vi "GetEndpointInfo.vi"(7 "LabVIEW Web Service Request":refnum<class "Web Request.lvclass">) -> ()   [LabVIEW 2017]
uses:
  <vilib>/wsapi/Web Request.lvclass
  JsonableWirelessEndpoint.ctl
  JsonableWirelessChannel.ctl
  <vilib>/addons/InsightCM/Devices/Shared/Ble/BleComm/BleComm.lvlib
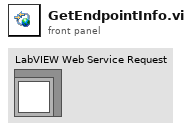
[diagram p1: front panel]
types:
  T1 = typedef "BleComm.lvlib/Endpoint.ctl" = cluster{"Serial Number":u64, "Ble Address":string, "Endpoint Type":T2, "Firmware Version":string, "Ignore Firmware":bool, "Firmware Recovery Mode":bool, "Password":string, "New Password":string, "Config Version":i32, "Sensor Group Id":string, "State":T3, "Acquiring":bool, "Acquisition Start Time":timestamp, "Ignore Gate":bool, "Sample Rate":T4, "Samples to Read":u32, "Last Communication":timestamp, "Last Acquisition":timestamp, "State Change":timestamp, "Last Status":timestamp, "Endpoint Busy Count":i32, "Properties":T5[], "Channels":T6[], "Gate":T7, "Error Timestamps":timestamp[]}
  T2 = typedef "BleComm.lvlib/Type.ctl" = enum16{"Gateway", "Spider", "Bluenose"}
  T3 = typedef "BleComm.lvlib/EndpointState.ctl" = enum16{"Unknown", "Discovered", "Bond Requested", "Bonded", "Firmware Version Requested", "Firmware Version Received", "Firmware Update Requested", "Firmware Ok", "Change Password Requested", "Password Ok", "Radio Update Requested", "Radio Ok", "Configure Requested", "Configured", "Error", "Error - Unbonding", "Error - Unknown", "Error - Quarantined"}
  T4 = typedef "Bluetooth Sensing.lvlib/SampleRate.ctl" = enum16{"25.6 kHz", "12.8 kHz", "6.4 kHz", "3.2 kHz", "1.6 kHz", "800 Hz"}
  T5 = typedef "KeyValuePair.ctl" = cluster{"Key":string, "Value":string}
  T6 = typedef "BleComm.lvlib/WirelessChannel.ctl" = cluster{"Channel Number":i32, "AssetId":string, "Sensor Type":string, "Mode":enum16{"Off", "Averaged", "Waveform"}, "Sensitivity":dbl, "Offset":dbl, "IEPE":enum16{"4 mA", "3 mA", "Off", "2 mA"}, "Coupling":enum16{"AC w/10 Hz cutoff", "AC w/2 Hz cutoff", "DC"}, "Unit":string, "Sw Ac Coupling":bool}
  T7 = typedef "BleComm.lvlib/Gate.ctl" = cluster{"Channel":u8, "Feature":string, "Level (EU)":dbl, "Properties":variant}
  T8 = typedef "JsonableWirelessEndpoint.ctl" = cluster{"Serial Number":string, "State":string, "Ble address":string, "Endpoint Type":string, "Firmware Version":string, "Password":string, "New Password":string, "Config Version":i32, "Sensor Group Id":string, "Acquisition Start Time":string, "Last Communication":string, "Last Acquisition":string, "State Change":string, "Endpoint Busy Count":i32, "Sample Rate":string, "Samples to Read":u32, "Properties":cluster{"Key":string, "Value":string}[], "Channels":T9[], "Gate Channel":u8, "Gate Feature":string, "Gate Level (EU)":dbl, "Error Timestamps":string[]}
  T9 = typedef "JsonableWirelessChannel.ctl" = cluster{"Channel Number":i32, "Type":string, "Sensitivity":dbl, "Offset":dbl, "IEPE":string, "Coupling":string, "Unit":string, "Sw Ac Coupling":bool}
  T10 = enum16{"AC w/10 Hz cutoff", "AC w/2 Hz cutoff", "DC"}
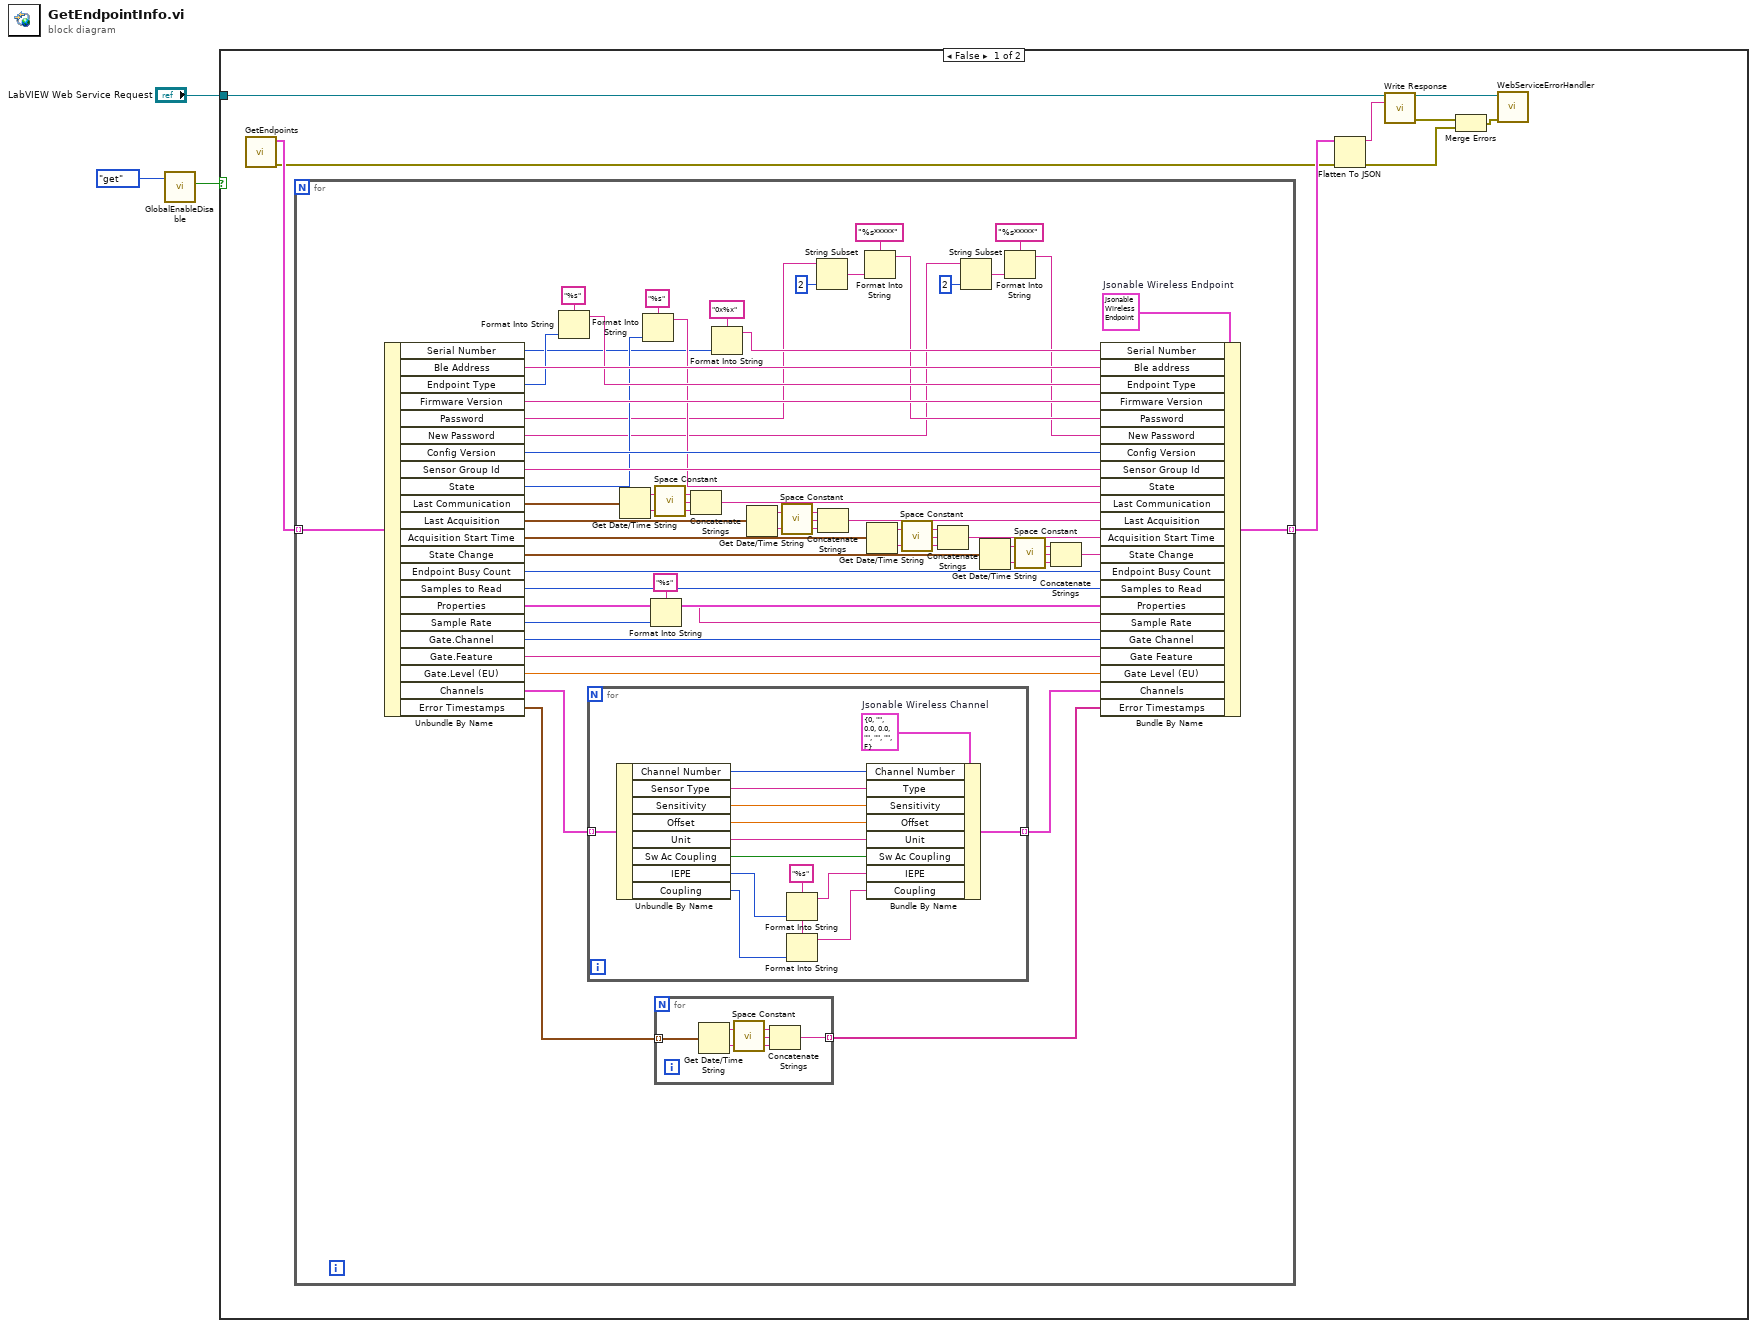
[diagram p0: block diagram]
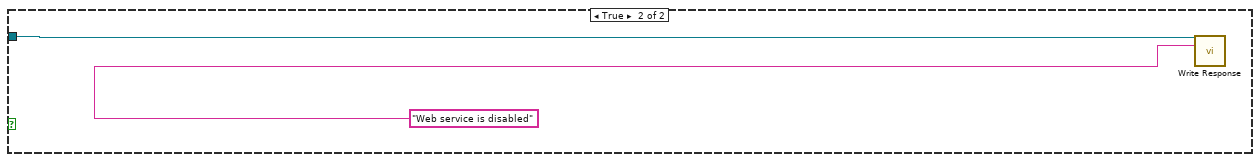
[diagram p2: hidden frame]
diagram:
  n1 = call "GlobalEnableDisable.vi"("action"=enum16{"init", "set", "get"}."get") -> ("DisableDeviceWebService"=w1:bool)  [unwired: 10 in]
  n2 = case shown="False" w1 {
    tunnel: "LabVIEW Web Service Request" -> [w12 w91]
    frame False {
      n3 = call <vilib>:"GetEndpoints.vi"() -> ("error out"=w4:errorcluster, "endpoints"=w5:T1[])  [unwired: 10 in]
      n4 = for {
        tunnel: w5 -> [w71] mode=indexing
        tunnel: [w65] -> w6 mode=indexing
        w70 = T8 {"Serial Number"="", "State"="", "Ble address"="", "Endpoint Type"="", "Firmware Version"="", "Password"="", "New Password"="", "Config Version"=0, "Sensor Group Id"="", "Acquisition Start Time"="", "Last Communication"="", "Last Acquisition"="", "State Change"="", "Endpoint Busy Count"=0, "Sample Rate"="", "Samples to Read"=0, "Properties"=[], "Channels"=[], "Gate Channel"=0, "Gate Feature"="", "Gate Level (EU)"=0.0, "Error Timestamps"=[]}  # Jsonable Wireless Endpoint
        n5 = Unbundle By Name(w71) -> ("Serial Number"=w24:u64, "Ble Address"=w46:string, "Endpoint Type"=w45:T2, "Firmware Version"=w43:string, "Password"=w18:string, "New Password"=w14:string, "Config Version"=w42:i32, "Sensor Group Id"=w41:string, "State"=w40:T3, "Last Communication"=w64:timestamp, "Last Acquisition"=w52:timestamp, "Acquisition Start Time"=w50:timestamp, "State Change"=w33:timestamp, "Endpoint Busy Count"=w38:i32, "Samples to Read"=w59:u32, "Properties"=w69:T5[], "Sample Rate"=w67:T4, "Gate.Channel"=w32:u8, "Gate.Feature"=w31:string, "Gate.Level (EU)"=w30:dbl, "Channels"=w29:T6[], "Error Timestamps"=w27:timestamp[])
        n6 = Format Into String(format string="%s", w45) -> (resulting string=w44:string)  [unwired: 2 in, 1 out]
        n7 = for {
          tunnel: w29 -> [w90] mode=indexing
          tunnel: [w77] -> w28 mode=indexing
          w84 = "%s" ("format string")
          w89 = T9 {"Channel Number"=0, "Type"="", "Sensitivity"=0.0, "Offset"=0.0, "IEPE"="", "Coupling"="", "Unit"="", "Sw Ac Coupling"=FALSE}  # Jsonable Wireless Channel
          n8 = Unbundle By Name(w90) -> ("Channel Number"=w88:i32, "Sensor Type"=w87:string, "Sensitivity"=w86:dbl, "Offset"=w85:dbl, "Unit"=w83:string, "Sw Ac Coupling"=w82:bool, "IEPE"=w81:enum16{"4 mA", "3 mA", "Off", "2 mA"}, "Coupling"=w79:T10)
          n9 = Format Into String(format string=w84, w81) -> (resulting string=w80:string)  [unwired: 2 in, 1 out]
          n10 = Format Into String(format string=w84, w79) -> (resulting string=w78:string)  [unwired: 2 in, 1 out]
          n11 = Bundle By Name(cluster=w89, "Channel Number"=w88, "Type"=w87, "Sensitivity"=w86, "Offset"=w85, "Unit"=w83, "Sw Ac Coupling"=w82, "IEPE"=w80, "Coupling"=w78) -> (w77:T9)
        }
        n12 = Get Date/Time String(seconds (now)=w64) -> (date string=w63:string, time string=w62:string)  [unwired: 2 in]
        n13 = Format Into String(format string="%s", w40) -> (resulting string=w39:string)  [unwired: 2 in, 1 out]
        n14 = Format Into String(format string="%s", w67) -> (resulting string=w66:string)  [unwired: 2 in, 1 out]
        n15 = call <vilib>:"Space Constant.vi"() -> ("String"=w61:string)
        n16 = for {
          tunnel: w27 -> [w74] mode=indexing
          tunnel: [w72] -> w26 mode=indexing
          n17 = Get Date/Time String(seconds (now)=w74) -> (date string=w76:string, time string=w73:string)  [unwired: 2 in]
          n18 = call <vilib>:"Space Constant.vi"() -> ("String"=w75:string)
          n19 = Concatenate Strings(w76, w75, w73) -> (w72:string)
        }
        n20 = Concatenate Strings(w63, w61, w62) -> (w60:string)
        n21 = Format Into String(format string="0x%x", w24) -> (resulting string=w23:string)  [unwired: 2 in, 1 out]
        n22 = Get Date/Time String(seconds (now)=w52) -> (date string=w56:string, time string=w57:string)  [unwired: 2 in]
        n23 = call <vilib>:"Space Constant.vi"() -> ("String"=w58:string)
        n24 = String Subset(string=w18, length (rest)=2 ("length (rest)")) -> (substring=w20:string)  [unwired: 1 in]
        n25 = Concatenate Strings(w56, w58, w57) -> (w51:string)
        n26 = Format Into String(format string="%s*****", w20) -> (resulting string=w17:string)  [unwired: 2 in, 1 out]
        n27 = Get Date/Time String(seconds (now)=w50) -> (date string=w55:string, time string=w54:string)  [unwired: 2 in]
        n28 = call <vilib>:"Space Constant.vi"() -> ("String"=w53:string)
        n29 = Concatenate Strings(w55, w53, w54) -> (w49:string)
        n30 = String Subset(string=w14, length (rest)=2 ("length (rest)")) -> (substring=w15:string)  [unwired: 1 in]
        n31 = Get Date/Time String(seconds (now)=w33) -> (date string=w35:string, time string=w36:string)  [unwired: 2 in]
        n32 = Format Into String(format string="%s*****", w15) -> (resulting string=w13:string)  [unwired: 2 in, 1 out]
        n33 = call <vilib>:"Space Constant.vi"() -> ("String"=w37:string)
        n34 = Concatenate Strings(w35, w37, w36) -> (w34:string)
        n35 = Bundle By Name(cluster=w70, "Serial Number"=w23, "Ble address"=w46, "Endpoint Type"=w44, "Firmware Version"=w43, "Password"=w17, "New Password"=w13, "Config Version"=w42, "Sensor Group Id"=w41, "State"=w39, "Last Communication"=w60, "Last Acquisition"=w51, "Acquisition Start Time"=w49, "State Change"=w34, "Endpoint Busy Count"=w38, "Samples to Read"=w59, "Properties"=w69, "Sample Rate"=w66, "Gate Channel"=w32, "Gate Feature"=w31, "Gate Level (EU)"=w30, "Channels"=w28, "Error Timestamps"=w26) -> (w65:T8)
      }
      n36 = Flatten To JSON(anything=w6, error in (no error)=w4) -> (JSON string=w7:string, 11:w8:errorcluster)  [unwired: 1 in]
      n37 = call <vilib>:"Write Response.vi"("LabVIEW Web Service Request"=w12, "response string"=w7) -> ("LabVIEW Web Service Request out"=w11:refnum<class "Web Request.lvclass">, "error out"=w10:errorcluster)  [unwired: 12 in]
      n38 = Merge Errors(w10, w8) -> (w9:errorcluster)
      n39 = call "WebServiceErrorHandler.vi"("LabVIEW Web Service Request"=w11, "error in (no error)"=w9) -> ()  [unwired: 12 in, 2 out]
    }
    frame True {
      n40 = call <vilib>:"Write Response.vi"("LabVIEW Web Service Request"=w91, "response string"="Web service is disabled") -> ()  [unwired: 12 in, 2 out]
    }
  }
